vi "csv to tdms.vi"(8 "error in (no error)":errorcluster, 10 "file path (dialog if empty)":path, 11 "device_type in":refnum<class "device_type.lvclass">) -> (0 "error out":errorcluster, 2 "raw PDW":u64[][](array[numeric]), 3 "device_type out":refnum<class "device_type.lvclass">)   [LabVIEW 2021, in "device_type.lvclass"]
uses:
  device_type.lvclass
  device_type.lvclass/device_type.ctl
  pulse_tx_vis/CTL/PDW_lv2.ctl
  pulse_tx_vis/CTL/mode_type.ctl
  78dac67b-a98c-4126-8064-665cba251dd6.vi
  <vilib>/Utility/file.llb/Read Delimited Spreadsheet (DBL).vi
  <vilib>/Comparison/Less/Less Functor/Less Functor.lvclass
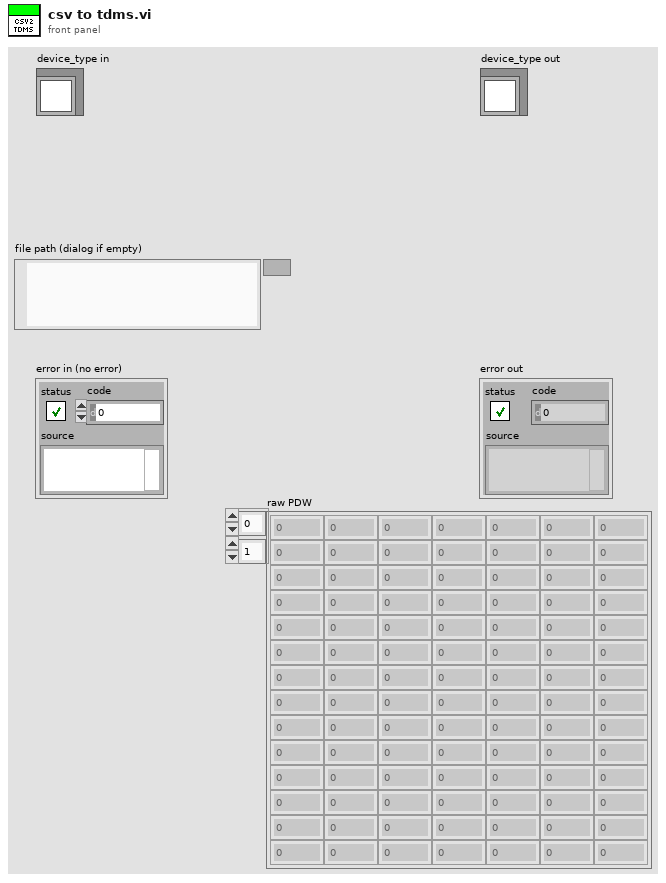
[diagram p1: front panel]
types:
  T1 = typedef "PDW_lv2.ctl" = cluster{"t start":dbl, "frequency (Hz)":dbl, "duration (sec)":dbl, "amp (lin)":dbl, "mod type":T2, "mod depth":dbl, "phase (rad)":dbl[]}
  T2 = typedef "mode_type.ctl" = enum8{"CW", "NC - CW", "NC - cw", "LFM", "BPSK", "QPSK"}
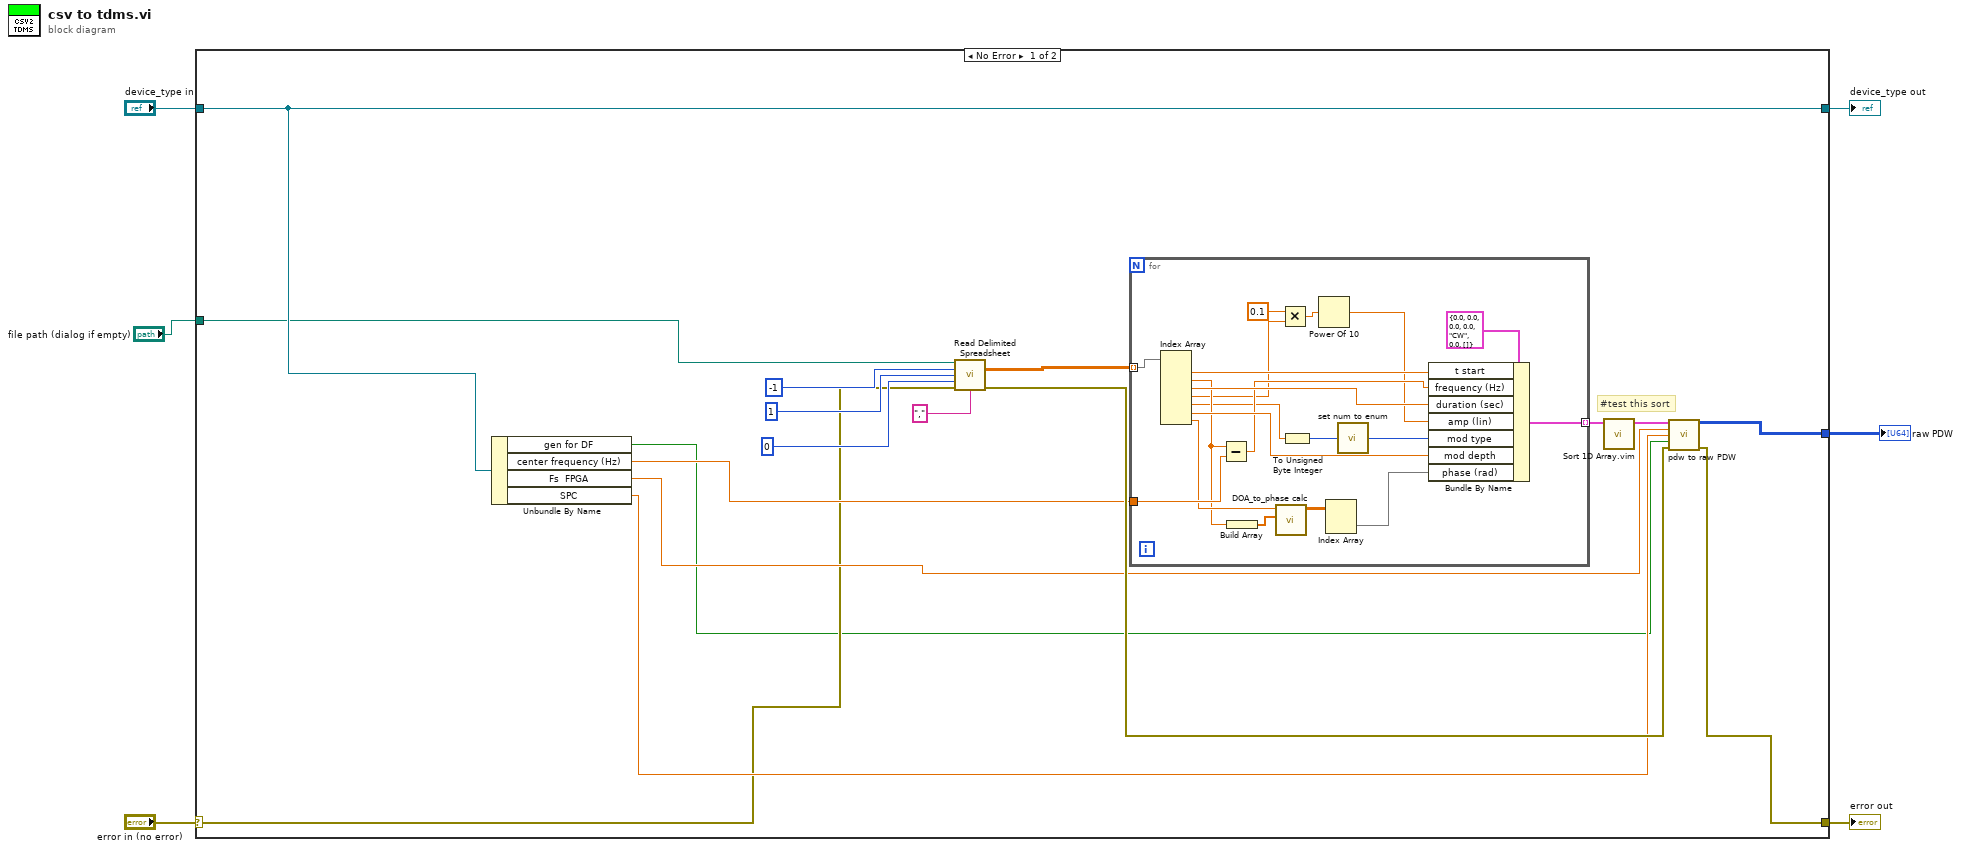
[diagram p0: block diagram]
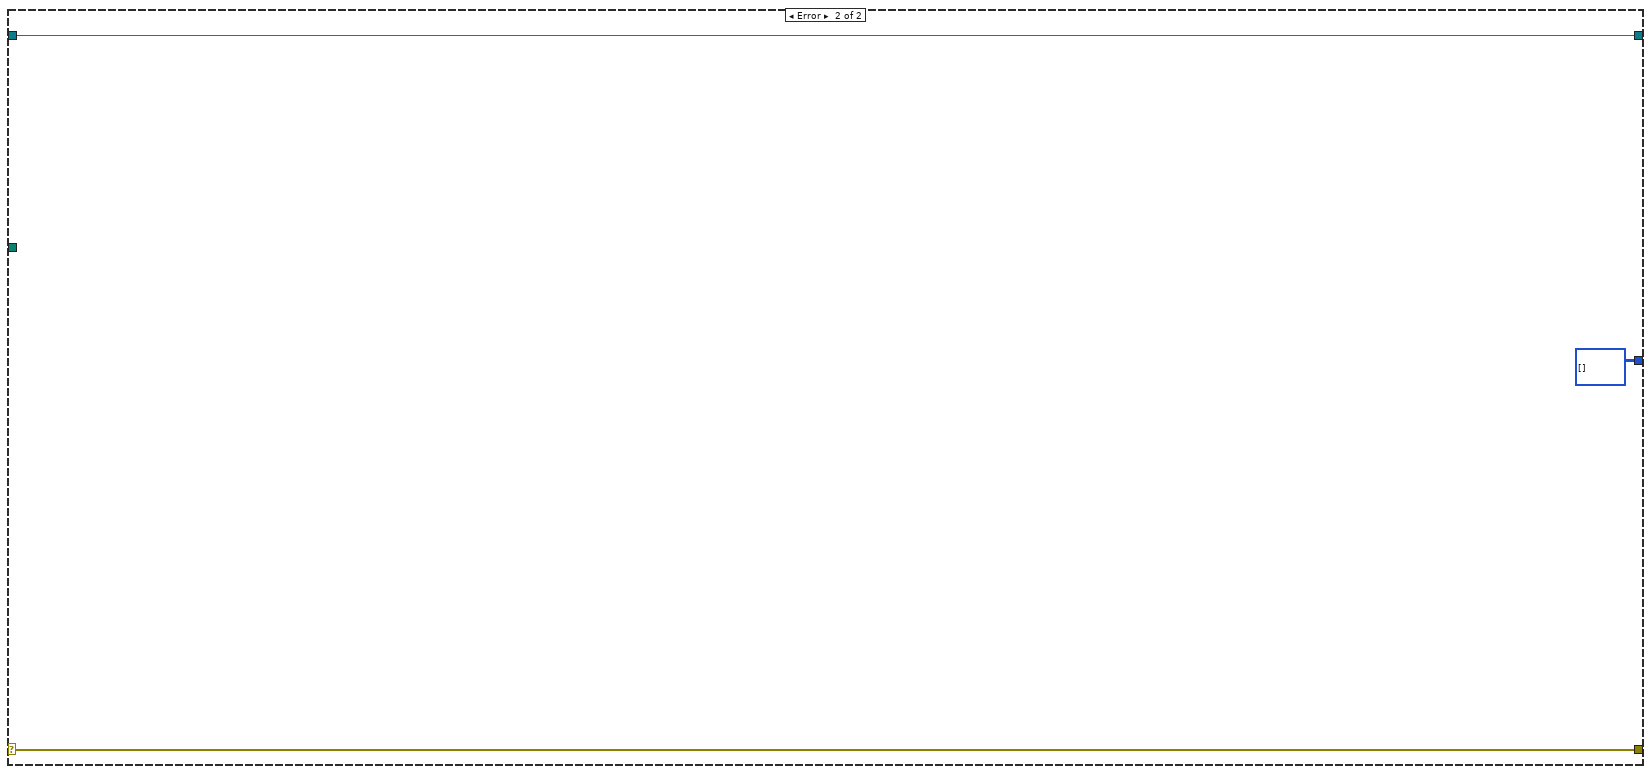
[diagram p2: hidden frame]
diagram:
  n1 = case shown="No Error" "error in (no error)" {
    selector: "error in (no error)" -> [w12 w46]
    tunnel: [w11 w46] -> w5
    tunnel: [w14 w45] -> w3
    tunnel: "device_type in" -> [w14 w45]
    tunnel: "file path (dialog if empty)" -> [w13 _]
    tunnel: [w10 u64[][] [] ("Array")] -> w1
    frame No Error {
      # "#test this sort"
      n2 = Unbundle By Name(w14) -> ("gen for DF"=w9:bool, "center frequency (Hz)"=w16:dbl, "Fs  FPGA"=w15:dbl, "SPC"=w17:dbl)
      n3 = call-poly <vilib>:"Read Delimited Spreadsheet.vi"("file path (dialog if empty)"=w13, "number of rows (all:-1)"=-1, "start of read offset (chars.:0)"=1, "max characters/row  (no limit:0)"=0, "error in (no error)"=w12, "delimiter (\\t)"="," ("delimiter (\\t)")) -> ("all rows"=w19:dbl[][], "error out"=w18:errorcluster)  [unwired: 4 in, 4 out]
      n4 = for {
        tunnel: [w42] -> w8 mode=indexing
        tunnel: w19 -> [w41] mode=indexing
        tunnel: w16 -> [w37]
        n5 = Index Array(array=w41) -> (element #1=w40:dbl, element #2=w34:dbl, element #3=w39:dbl, element #4=w30:dbl, element #5=w26:dbl, element #6=w38:dbl, element #7=w35:dbl)  [unwired: 7 in]
        n6 = Subtract(x=w34, y=w37) -> (x-y=w36:dbl)
        n7 = Build Array(w34) -> (w33:dbl[])
        n8 = call "DOA_to_phase calc.vi"("f set (Hz)"=w33, "DOA (deg)"=w35) -> ("phase (rad)"=w28:dbl[][])  [unwired: 9 in]
        n9 = Multiply(x=0.1, y=w30) -> (x*y=w31:dbl)
        n10 = To Unsigned Byte Integer(number=w26) -> (unsigned 8bit integer=w25:u8)
        n11 = Power Of 10(x=w31) -> (10^x=w29:dbl)
        n12 = Index Array(array=w28) -> (element=w27:dbl[])  [unwired: 2 in]
        n13 = call "set num to enum.vi"("Numeric in"=w25) -> ("Numeric out"=w24:T2)
        n14 = Bundle By Name(cluster=T1 {"t start"=0.0, "frequency (Hz)"=0.0, "duration (sec)"=0.0, "amp (lin)"=0.0, "mod type"=enum."CW", "mod depth"=0.0, "phase (rad)"=[]}, "t start"=w40, "frequency (Hz)"=w36, "duration (sec)"=w39, "amp (lin)"=w29, "mod type"=w24, "mod depth"=w38, "phase (rad)"=w27) -> (w42:T1)
      }
      n15 = call "Sort 1D Array.vim"("unsorted array"=w8) -> ("sorted array"=w7:T1[])  [unwired: 10 in]
      n16 = call "pdw to raw PDW.vi"("PDWs"=w7, "Fs fpGa"=w15, "SPC"=w17, "gen for DF"=w9, "erorr in"=w18) -> ("Array"=w10:u64[][], "erorr out"=w11:errorcluster)  [unwired: 8 in, 1 out]
    }
    frame Error {
    }
  }
  "error out" <- w5
  "device_type out" <- w3
  "raw PDW" <- w1
